vi "Graph Motion Profile Points.vi"(11 "Motion Profile Array":T1[](array[typedef])) -> (3 "Array":cluster{dbl[], dbl[]}[](array[cluster]))   [LabVIEW 2019]
uses:
  Motion Profile Generator/Type Defs/Motion Profile Point.ctl
  Motion Profile Generator/Motion Profile Generator.lvclass
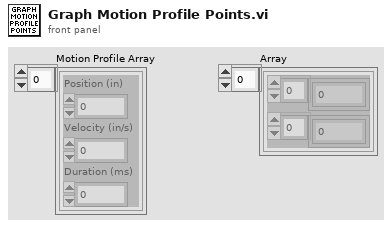
[diagram p1: front panel]
types:
  T1 = typedef "Motion Profile Generator.lvclass/Motion Profile Point.ctl" = cluster{"Position (in)":dbl, "Velocity (in/s)":dbl, "Duration (ms)":dbl}
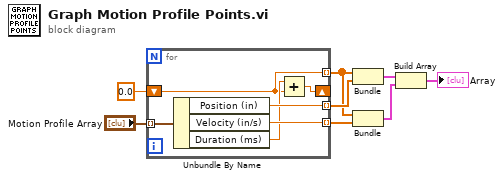
[diagram p0: block diagram]
diagram:
  n1 = for {
    tunnel: "Motion Profile Array" -> [w14] mode=indexing
    tunnel: [w13] -> w4 mode=indexing
    tunnel: [w12] -> w5 mode=indexing
    shift-right: [w10] -> _
    shift-left: 0.0 -> [w9]
    tunnel: [w9] -> w3 mode=indexing
    n2 = Unbundle By Name(w14) -> ("Position (in)"=w13:dbl, "Velocity (in/s)"=w12:dbl, "Duration (ms)"=w11:dbl)
    n3 = Add(x=w11, y=w9) -> (x+y=w10:dbl)
  }
  n4 = Bundle(w3, w4) -> (w6:cluster{dbl[], dbl[]})  [unwired: 1 in]
  n5 = Bundle(w3, w5) -> (w7:cluster{dbl[], dbl[]})  [unwired: 1 in]
  n6 = Build Array(w6, w7) -> (→"Array":cluster{dbl[], dbl[]}[])
